vi "ACQ MergeTempFiles.vi"(1 "Base file path amb comentaris":path, 2 "file sufix num. in":u32, 3 "Comptador events per file in":u32) -> (6 "file sufix num. out":u32, 7 "Comptador events per file out":u32)   [LabVIEW 2015, in "VIPM2.lvlib"]
doc: "ACQ DATA: merge temp files."
uses:
  VIPM2.lvlib
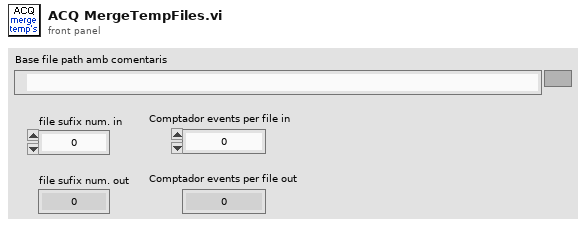
[diagram p1: front panel]
types:
  T1 = enum16{"open", "replace", "create", "open or create", "replace or create", "replace or create with confirmation"}
  T2 = enum16{"big-endian, network order", "native, host order", "little-endian"}
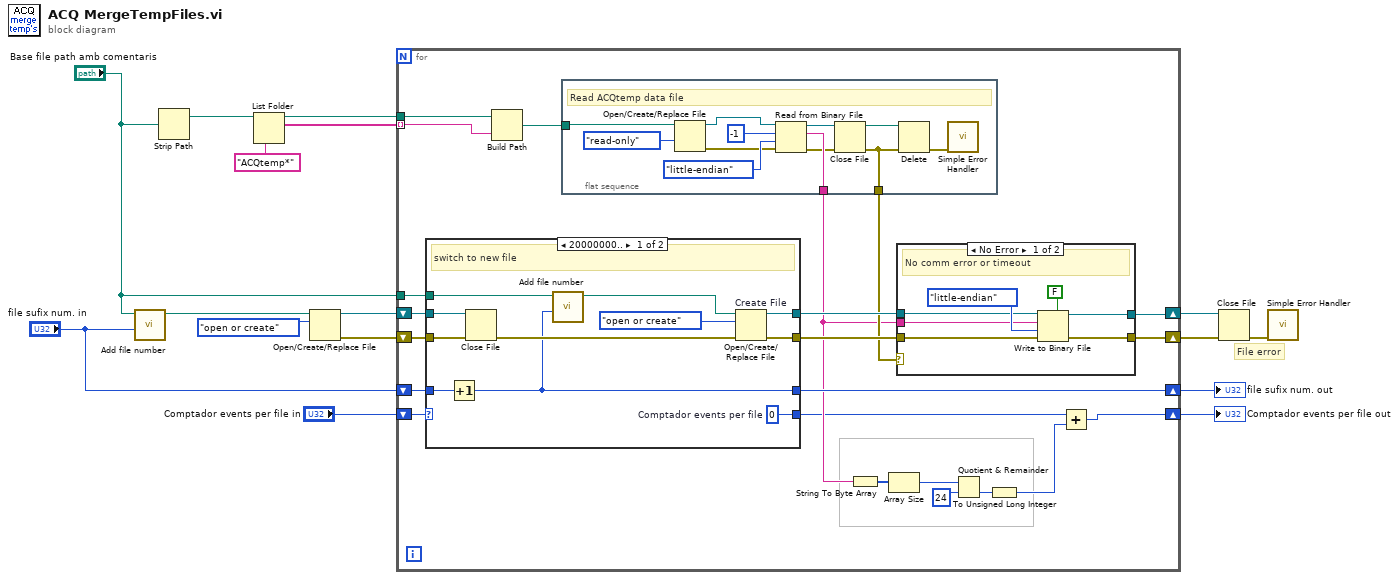
[diagram p0: block diagram]
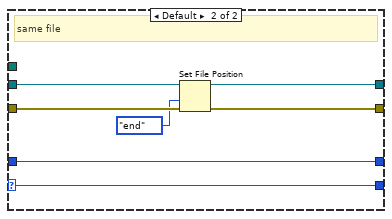
[diagram p3: hidden frame]
diagram:
  # "File error"
  n1 = call "Add file number.vi"("sufix number"="file sufix num. in", "file path"="Base file path amb comentaris") -> ("incremented file path"=w14:path)  [unwired: 9 in]
  n2 = Strip Path(path="Base file path amb comentaris") -> (stripped path=w15:path)  [unwired: 1 out]
  n3 = List Folder(path=w15, pattern="ACQtemp*") -> (path out=w11:path, filenames=w12:string[])  [unwired: 2 in, 2 out]
  n4 = Open/Create/Replace File(file path (use dialog)=w14, operation (0:open)=T1."open or create") -> (refnum out=w10:refnum<file>, error out=w9:errorcluster)  [unwired: 4 in, 1 out]
  n5 = for {
    tunnel: w12 -> [w37] mode=indexing
    tunnel: w11 -> [w38]
    tunnel: "Base file path amb comentaris" -> [w33]
    shift-right: [w30] -> w2
    shift-left: "file sufix num. in" -> [w32]
    shift-right: [w25] -> w4
    shift-left: w9 -> [w34]
    shift-right: [w17] -> w1
    shift-left: "Comptador events per file in" -> [w31]
    shift-right: [w26] -> w5
    shift-left: w10 -> [w35]
    n6 = case shown="20000000.." w31 {
      selector: w31 -> [_ w60]
      tunnel: w35 -> [w56 w65]
      tunnel: w34 -> [w57 w64]
      tunnel: [w50 w62] -> w28
      tunnel: [w51 w61] -> w29
      tunnel: [w58 w60] -> w20
      tunnel: [w48 w59] -> w30
      tunnel: w32 -> [w55 w59]
      tunnel: w33 -> [w54 _]
      frame 20000000.. {
        w58 = u32 0  # Comptador events per file
        # "switch to new file"
        n7 = Increment(x=w55) -> (x+1=w48:u32)
        n8 = Close File(refnum=w56, error in=w57) -> (error out=w49:errorcluster)  [unwired: 1 out]
        n9 = call "Add file number.vi"("sufix number"=w48, "file path"=w54) -> ("incremented file path"=w53:path)  [unwired: 9 in]
        n10 = Open/Create/Replace File "Create File"(file path (use dialog)=w53, error in=w49, operation (0:open)=T1."open or create") -> (refnum out=w51:refnum<file>, error out=w50:errorcluster)  [unwired: 3 in, 1 out]
      }
      frame Default {
        # "same file"
        n11 = Set File Position(refnum=w65, from (0:start)=enum16{"start", "end", "current"}."end", error in=w64) -> (refnum out=w61:refnum<file>, error out=w62:errorcluster)  [unwired: 1 in]
      }
    }
    n12 = Build Path(base path=w38, name or relative path=w37) -> (appended path=w36:path)
    n13 = flat-sequence {
      tunnel: [w77] -> w21
      tunnel: w36 -> [w69]
      tunnel: [w66] -> w27
      frame #0 {
        # "Read ACQtemp data file"
        n14 = Open/Create/Replace File(file path (use dialog)=w69, access (0:read/write)=enum16{"read/write", "read-only", "write-only"}."read-only") -> (refnum out=w71:refnum<file>, error out=w70:errorcluster)  [unwired: 4 in, 1 out]
        n15 = Read from Binary File(8:w70, 9:T2."little-endian" ("byte order (0:big-endian, network order)"), 10:-1 ("count"), 11:w71) -> (0:w73:errorcluster, 2:w77:string, 3:w74:refnum<file>)  [unwired: 2 in, 1 out]
        n16 = Close File(refnum=w74, error in=w73) -> (path=w67:path, error out=w66:errorcluster)
        n17 = Delete(path (use dialog)=w67, error in=w66) -> (error out=w68:errorcluster)  [unwired: 3 in, 2 out]
        n18 = call <vilib>:"Simple Error Handler.vi"("error in (no error)"=w68) -> ()  [unwired: 4 in, 5 out]
      }
    }
    n19 = String To Byte Array(string=w21) -> (unsigned byte array=w24:u8[])
    n20 = Array Size(array=w24) -> (size(s)=w23:i32)
    n21 = case shown="No Error" w27 {
      tunnel: [w43 w47] -> w26
      tunnel: [w42 w46] -> w25
      tunnel: w21 -> [w41 _]
      tunnel: w28 -> [w40 w46]
      tunnel: w29 -> [w39 w47]
      frame No Error {
        # "No comm error or timeout"
        n22 = Write to Binary File(file (use dialog)=w39, data=w41, error in=w40, 5:FALSE ("prepend array or string size? (T)"), 9:T2."little-endian" ("byte order (0:big-endian, network order)")) -> (refnum out=w43:refnum<file>, error out=w42:errorcluster)  [unwired: 1 in, 1 out]
      }
      frame Error {
      }
    }
    n23 = Quotient & Remainder(x=w23, y=24) -> (floor(x/y)=w19:i32)  [unwired: 1 out]
    n24 = To Unsigned Long Integer(number=w19) -> (unsigned 32bit integer=w18:u32)
    n25 = Add(x=w20, y=w18) -> (x+y=w17:u32)
  }
  "file sufix num. out" <- w2
  "Comptador events per file out" <- w1
  n26 = Close File(refnum=w5, error in=w4) -> (error out=w3:errorcluster)  [unwired: 1 out]
  n27 = call <vilib>:"Simple Error Handler.vi"("error in (no error)"=w3) -> ()  [unwired: 4 in, 5 out]
